vi "PathPlanner_PathFinder_Constants.vi"() -> (1 "EPS":dbl, 2 "SMOOTHING_CONTROL_PCT":dbl, 3 "SMOOTHING_ANCHOR_PCT":dbl)   [LabVIEW 2019, in "PathPlanner24.lvlib"]
doc: "Internal function. Not to be used by end users."
uses:
  PathPlanner24.lvlib
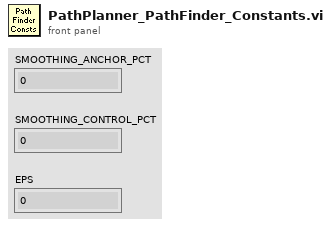
[diagram p1: front panel]
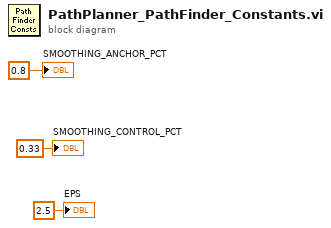
[diagram p0: block diagram]
diagram:
  "SMOOTHING_ANCHOR_PCT" <- 0.8 ("SMOOTHING_ANCHOR_PCT")
  "SMOOTHING_CONTROL_PCT" <- 0.33 ("SMOOTHING_CONTROL_PCT")
  "EPS" <- 2.5 ("EPS")
